vi "Source_Ctrl.vi"(4 "Error in":errorcluster, 5 "SourceGroup":u16, 6 "ON/OFF":bool=TRUE, 7 "VISA in":refnum<visa-resource-name>) -> (0 "error out":errorcluster, 3 "VISA out":refnum<visa-resource-name>)   [LabVIEW 2019]
uses:
  c4360b90-cf2e-4cfe-8423-d1d110129d18.vi
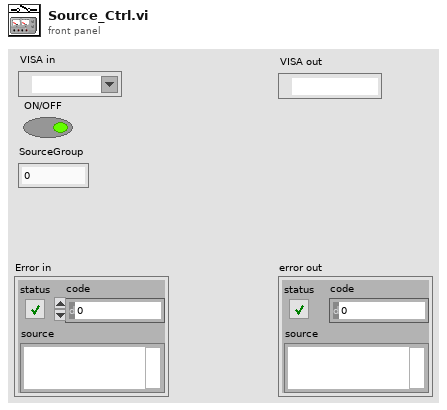
[diagram p1: front panel]
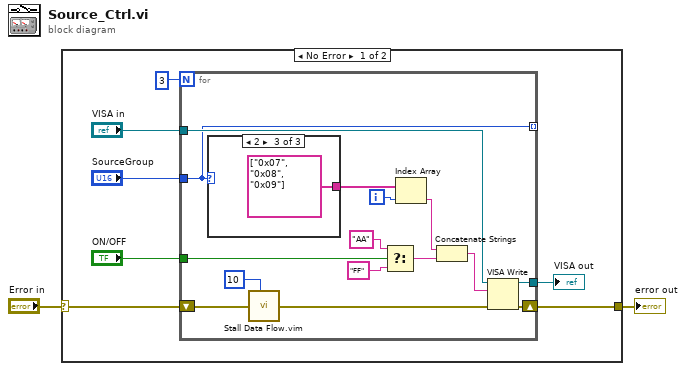
[diagram p0: block diagram]
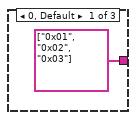
[diagram p2: hidden frame]
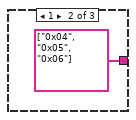
[diagram p3: hidden frame]
diagram:
  n1 = case shown="No Error" "Error in" {
    selector: "Error in" -> [w7 w28]
    tunnel: [w3 w28] -> w1
    frame No Error {
      n2 = for {
        N: 3 -> [_]
        tunnel: "VISA in" -> [w24]
        tunnel: [w13] -> _ mode=indexing
        tunnel: [w22] -> w4
        tunnel: "ON/OFF" -> [w14]
        tunnel: "SourceGroup" -> [w13]
        shift-right: [w23] -> w3
        shift-left: w7 -> [w11]
        i -> [w21]
        n3 = case shown="2" w13 {
          tunnel: [string[] ["0x01", "0x02", "0x03"] string[] ["0x04", "0x05", "0x06"] string[] ["0x07", "0x08", "0x09"]] -> w20
          frame 0, Default {
          }
          frame 1 {
          }
          frame 2 {
          }
        }
        n4 = call "Stall Data Flow.vim"("value in"=w11, "milliseconds to wait"=u32 10) -> ("value out"=w10:errorcluster)  [unwired: 1 out]
        n5 = Select(t="AA", s=w14, f="FF") -> (s? t:f=w16:string)
        n6 = Index Array(array=w20, index=w21) -> (element=w19:string)
        n7 = Concatenate Strings(w19, w16) -> (w15:string)
        n8 = VISA Write(VISA resource name=w24, write buffer=w15, error in (no error)=w10) -> (VISA resource name out=w22:refnum<visa-resource-name>, error out=w23:errorcluster)  [unwired: 1 out]
      }
      "VISA out" <- w4
    }
    frame Error {
    }
  }
  "error out" <- w1
